vi "lqManifestation.vi"(8 "error in (no error)":errorcluster, 11 "QObject in":refnum<class "QObject.lvclass">) -> (0 "error out":errorcluster, 2 "Manifestation":u32, 3 "QObject out":refnum<class "QObject.lvclass">)   [LabVIEW 2013, in "Template.lvlib" / "QObject.lvclass"]
uses:
  QObject.lvclass
  QObject.lvclass/QObject.ctl
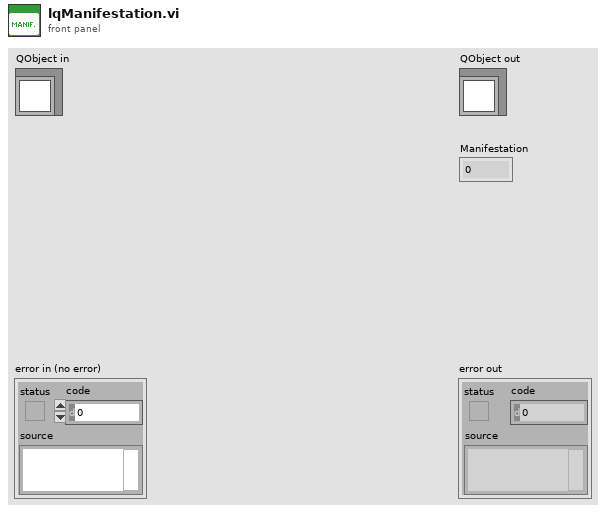
[diagram p1: front panel]
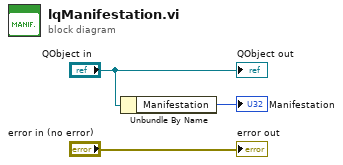
[diagram p0: block diagram]
diagram:
  n1 = Unbundle By Name("QObject in") -> ("Manifestation"=→"Manifestation":u32)
  "error out" <- "error in (no error)"
  "QObject out" <- "QObject in"
